vi "3D Gcode simulator.vi"() -> ()   [LabVIEW 2020]
uses:
  <vilib>/Native 3D Graph/xcontrol/3DPC_SurfacePlot.xctl
panel:
  out "3D Graph":refnum<class "Base Datatype.lvclass">[](xcontrol)
  out "XY Graph":cluster{"X":dbl, "Y":dbl}[](graph)
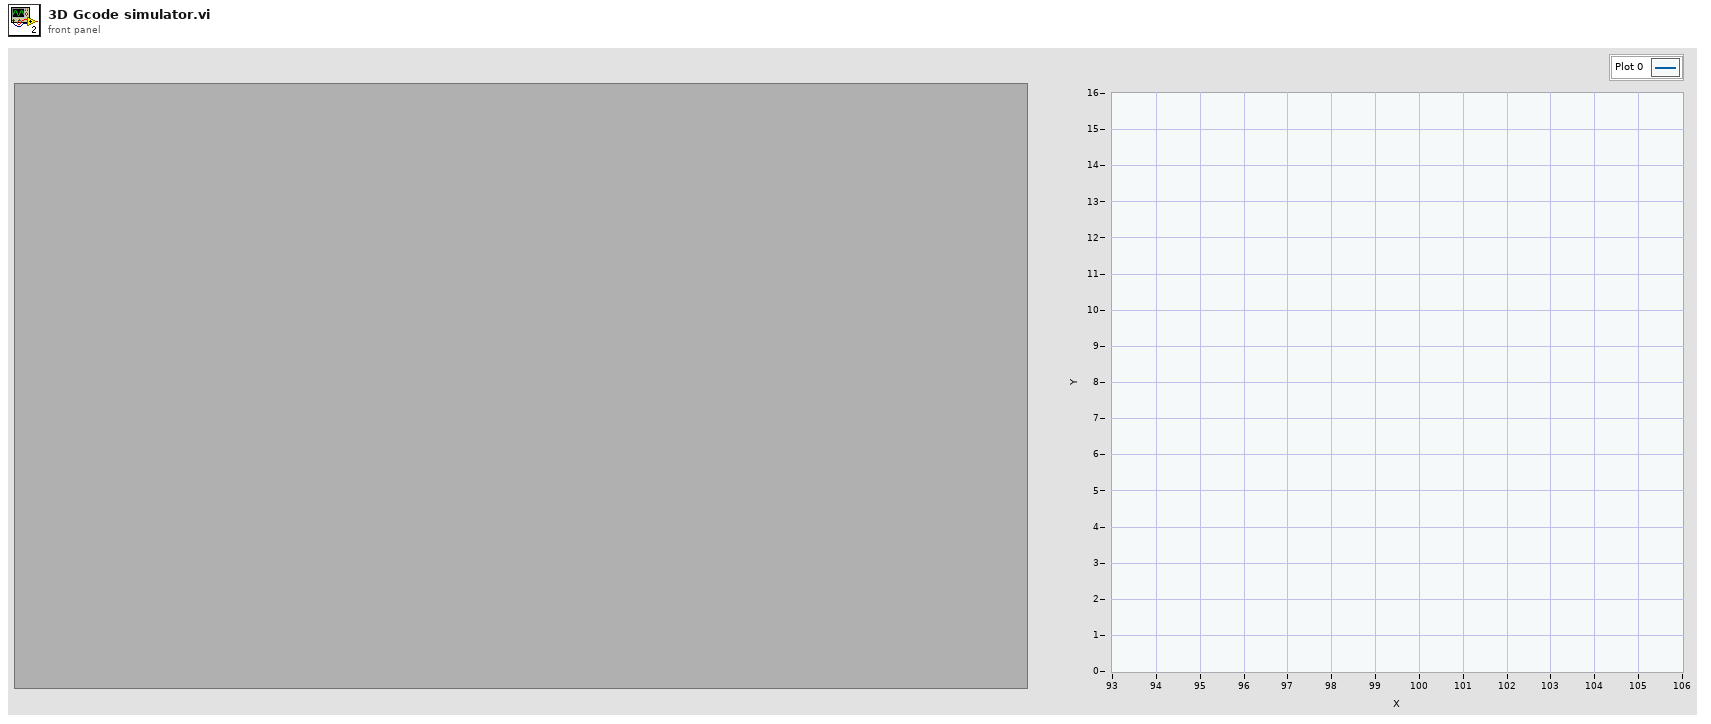
[diagram p1: front panel]
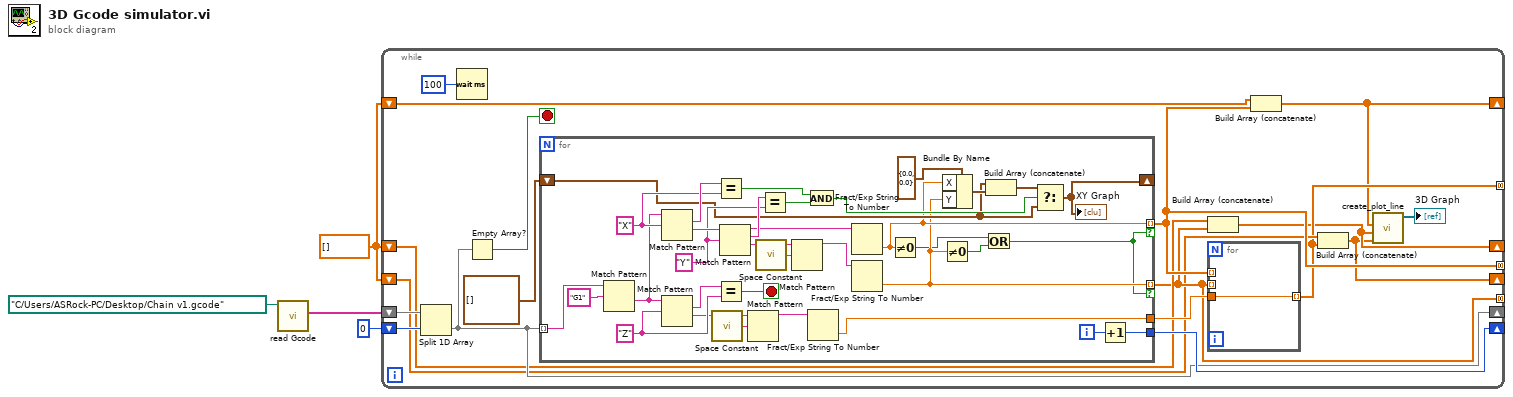
[diagram p0: block diagram]
diagram:
  w1 = dbl[] []
  n1 = call "read Gcode.vi"("Gcode path (use dialog)"=path "C:/Users/ASRock-PC/Desktop/Chain v1.gcode") -> ("Gcode Array"=w4:string[])  [unwired: 8 in, 2 out]
  n2 = while {
    shift-right: [w22] -> _
    shift-left: 0 -> [w20]
    shift-right: [w18] -> _
    shift-left: w4 -> [w21]
    tunnel: [w14] -> _ mode=concatenating
    tunnel: [w12] -> _ mode=concatenating
    tunnel: [w10] -> _ mode=concatenating
    shift-right: [w9] -> _
    shift-left: w1 -> [w15]
    shift-right: [w8] -> _
    shift-left: w1 -> [w13]
    shift-right: [w7] -> _
    shift-left: w1 -> [w11]
    stop <- w19 stop-if-true
    n3 = Split 1D Array(array=w21, index=w20) -> (second subarray=w18:string[])  [unwired: 1 out]
    n4 = Wait (ms)(milliseconds to wait=u32 100) -> ()  [unwired: 1 out]
    n5 = Empty Array?(array=w18) -> (empty?=w19:bool)
    n6 = for {
      tunnel: w18 -> [w57] mode=indexing
      tunnel: [w39] -> w22
      shift-right: [w34] -> _
      shift-left: cluster{"X":dbl, "Y":dbl}[] [] ("XY Graph 2") -> [w35]
      tunnel: [w33] -> w14 mode=indexing if=w24
      tunnel: [w32] -> w12 mode=indexing if=w24
      tunnel: [w26] -> w16
      i -> [w40]
      stop <- w41 stop-if-true
      w42 = "Z" ("regular expression")
      w49 = "Y" ("regular expression")
      w51 = "X" ("regular expression")
      n7 = Match Pattern(string=w57, regular expression="G1") -> (after substring=w25:string)  [unwired: 1 in, 3 out]
      n8 = Match Pattern(string=w25, regular expression=w51) -> (match substring=w52:string, after substring=w55:string)  [unwired: 1 in, 2 out]
      n9 = Match Pattern(string=w25, regular expression=w42) -> (match substring=w43:string, after substring=w28:string)  [unwired: 1 in, 2 out]
      n10 = call <vilib>:"Space Constant.vi"() -> ("String"=w29:string)
      n11 = Equal?(x=w52, y=w51) -> (x = y?=w48:bool)
      n12 = Equal?(x=w43, y=w42) -> (x = y?=w41:bool)
      n13 = Match Pattern(string=w55, regular expression=w49) -> (before substring=w46:string, match substring=w50:string, after substring=w54:string)  [unwired: 1 in, 1 out]
      n14 = Match Pattern(string=w28, regular expression=w29) -> (before substring=w27:string)  [unwired: 1 in, 3 out]
      n15 = call <vilib>:"Space Constant.vi"() -> ("String"=w53:string)
      n16 = Equal?(x=w50, y=w49) -> (x = y?=w47:bool)
      n17 = Match Pattern(string=w54, regular expression=w53) -> (before substring=w45:string)  [unwired: 1 in, 3 out]
      n18 = And(x=w48, y=w47) -> (x .and. y?=w38:bool)
      n19 = Fract/Exp String To Number(string=w27) -> (number=w26:dbl)  [unwired: 3 in, 1 out]
      n20 = Fract/Exp String To Number(string=w46) -> (number=w33:dbl)  [unwired: 3 in, 1 out]
      n21 = Fract/Exp String To Number(string=w45) -> (number=w32:dbl)  [unwired: 3 in, 1 out]
      n22 = Not Equal To 0?(x=w33) -> (x != 0?=w31:bool)
      n23 = Not Equal To 0?(x=w32) -> (x != 0?=w30:bool)
      n24 = Bundle By Name(cluster=cluster{"X":dbl, "Y":dbl} {"X"=0.0, "Y"=0.0} ("XY Graph"), "X"=w33, "Y"=w32) -> (w36:cluster{"X":dbl, "Y":dbl})
      n25 = Or(x=w31, y=w30) -> (x .or. y?=w24:bool)
      n26 = Build Array (concatenate)(w35, w36) -> (w37:cluster{"X":dbl, "Y":dbl}[])
      n27 = Select(t=w37, s=w38, f=w35) -> (s? t:f=w34:cluster{"X":dbl, "Y":dbl}[])
      "XY Graph" <- w34
      n28 = Increment(x=w40) -> (x+1=w39:i32)
    }
    n29 = Build Array (concatenate)(w13, w12) -> (w8:dbl[])
    n30 = for {
      tunnel: w14 -> [_] mode=indexing
      tunnel: w12 -> [_] mode=indexing
      tunnel: [w23] -> w10 mode=indexing
      tunnel: w16 -> [w23]
    }
    n31 = Build Array (concatenate)(w15, w14) -> (w9:dbl[])
    n32 = Build Array (concatenate)(w11, w10) -> (w7:dbl[])
    n33 = call <vilib>:"create_plot_line.vi"("z vector"=w7, "y vector"=w8, "x vector"=w9) -> ("plots out"=→"3D Graph":refnum<class "Base Datatype.lvclass">[])  [unwired: 2 in, 6 out]
  }
